vi "TimingGenFXP_src.vi"(0 "Upercent":fxp<+/-,32,4> caption="u voltage", 1 "Period":u32, 5 "Vpercent":fxp<+/-,32,4> caption="v voltage", 7 "Wpercent":fxp<+/-,32,4> caption="w voltage") -> (4 "U_Timing":T1, 6 "V_Timing":T1, 8 "W_timing":T1)   [LabVIEW 2015]
uses:
  ON_OFF_timing.ctl
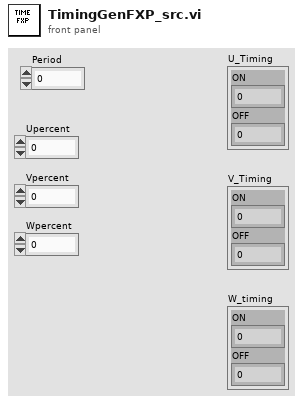
[diagram p1: front panel]
types:
  T1 = typedef "ON_OFF_timing.ctl" = cluster{"ON":u32, "OFF":u32}
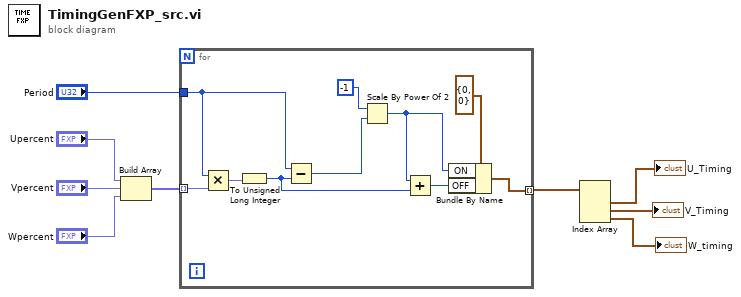
[diagram p0: block diagram]
diagram:
  n1 = Build Array("Upercent", "Vpercent", "Wpercent") -> (w6:fxp<+/-,32,4>[])
  n2 = for {
    tunnel: w6 -> [w19] mode=indexing
    tunnel: "Period" -> [w15]
    tunnel: [w17] -> w4 mode=indexing
    n3 = Multiply(x=w15, y=w19) -> (x*y=w16:fxp<+/-,64,36>)
    n4 = To Unsigned Long Integer(number=w16) -> (unsigned 32bit integer=w12:u32)
    n5 = Subtract(x=w15, y=w12) -> (x-y=w10:u32)
    n6 = Scale By Power Of 2(n=i16 -1, x=w10) -> (x*2^n=w13:u32)
    n7 = Add(x=w13, y=w12) -> (x+y=w11:u32)
    n8 = Bundle By Name(cluster=T1 {"ON"=0, "OFF"=0} ("ON_OFF"), "ON"=w13, "OFF"=w11) -> (w17:T1)
  }
  n9 = Index Array(array=w4) -> (element #1=→"U_Timing":T1, element #2=→"V_Timing":T1, element #3=→"W_timing":T1)  [unwired: 3 in]
